vi "Gen_Simulated_Data.vi"(8 "error in (no error)":errorcluster) -> (0 "error out":errorcluster, 2 "Sinal Frequencia":dbl[](graph), 3 "Sinal Tempo":cluster{"t0":dbl, "dt":dbl, "Y":dbl[]}(graph))   [LabVIEW 2019]
uses:
  <vilib>/addons/Modulation/Analog/controls/Complex Data Waveform.ctl
  <vilib>/addons/Modulation/niAMT.lvlib
  <vilib>/Analysis/NI_AALPro.lvlib
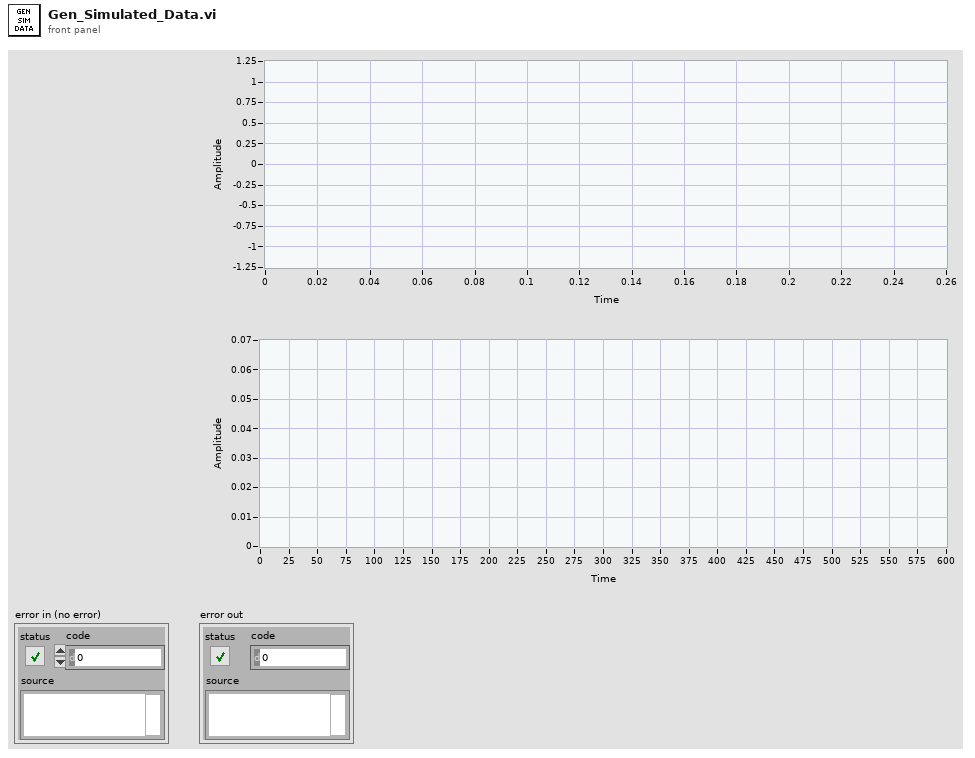
[diagram p1: front panel]
types:
  T1 = typedef "niAMT.lvlib/Complex Data Waveform.ctl" = cluster{"t0":dbl, "dt":dbl, "Y":cdb[]}
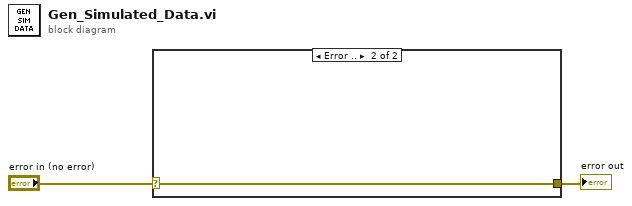
[diagram p0: block diagram]
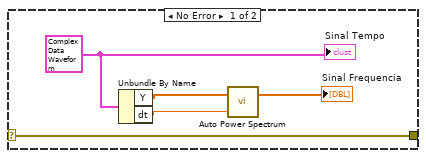
[diagram p2: hidden frame]
diagram:
  n1 = case shown="Error .." "error in (no error)" {
    selector: "error in (no error)" -> [w3 w8]
    tunnel: [w3 w8] -> w2
    frame No Error {
      w6 = T1 {"t0"=0.0, "dt"=3.6231884057971014e-05, "Y"=array[6970 elements]} ("output complex waveform")
      n2 = Unbundle By Name(w6) -> ("Y"=w4:cdb[], "dt"=w5:dbl)
      n3 = call <vilib>:"Auto Power Spectrum.vi"("dt"=w5, "Signal (V)"=w4) -> ("Power Spectrum (V^2 rms)"=→"Sinal Frequencia":dbl[])  [unwired: 1 out]
      "Sinal Tempo" <- w6
    }
    frame Error {
    }
  }
  "error out" <- w2
